vi "Hatch Pannel Test.vi"(10 "Run?":bool) -> ()   [LabVIEW 2018]
uses:
  SubSystems/Hatch Panel Intake/Hatch Panel Intake Global.vi
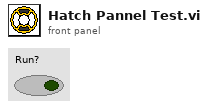
[diagram p1: front panel]
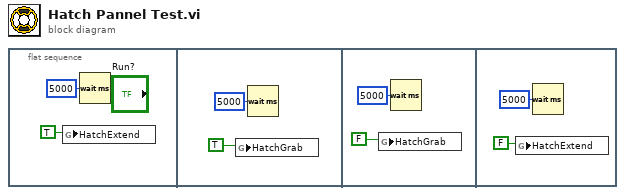
[diagram p0: block diagram]
diagram:
  n1 = flat-sequence {
    frame #0 {
      n2 = global write "Hatch Panel Intake Global.vi" "HatchExtend"(TRUE) -> ()
      n3 = Wait (ms)(milliseconds to wait=u32 5000) -> ()  [unwired: 1 out]
    }
    frame #1 {
      n4 = global write "Hatch Panel Intake Global.vi" "HatchGrab"(TRUE) -> ()
      n5 = Wait (ms)(milliseconds to wait=u32 5000) -> ()  [unwired: 1 out]
    }
    frame #2 {
      n6 = global write "Hatch Panel Intake Global.vi" "HatchGrab"(FALSE) -> ()
      n7 = Wait (ms)(milliseconds to wait=u32 5000) -> ()  [unwired: 1 out]
    }
    frame #3 {
      n8 = global write "Hatch Panel Intake Global.vi" "HatchExtend"(FALSE) -> ()
      n9 = Wait (ms)(milliseconds to wait=u32 5000) -> ()  [unwired: 1 out]
    }
  }
